vi "Load.vi"(8 "error in (no error)":errorcluster, 10 "Path":path, 11 "CNN in":refnum<class "CNN.lvclass">) -> (0 "error out":errorcluster, 3 "CNN out":refnum<class "CNN.lvclass">)   [LabVIEW 2016, in "CNN.lvclass"]
uses:
  CNN.lvclass
  CNN.lvclass/CNN.ctl
  <vilib>/Utility/file.llb/Read Delimited Spreadsheet (DBL).vi
panel:
  out "PFPC":i32[](array[numeric])
  out "all rows":dbl[][](array[numeric])
  out "size(s)":i32
  out "No Pre":i32[](array[numeric])
  out "Pre Ids":i32[](array[numeric])
  out "NoN":i32[](array[numeric])
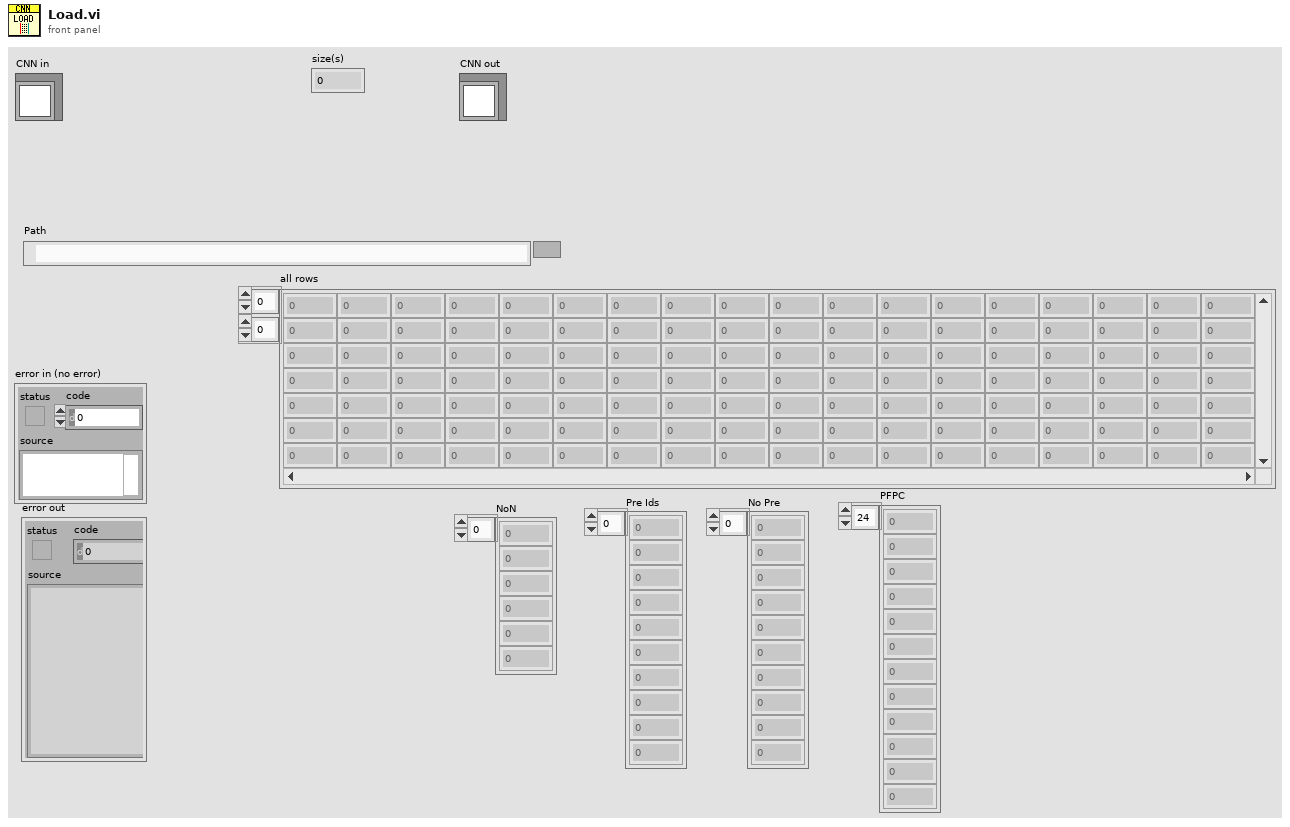
[diagram p1: front panel]
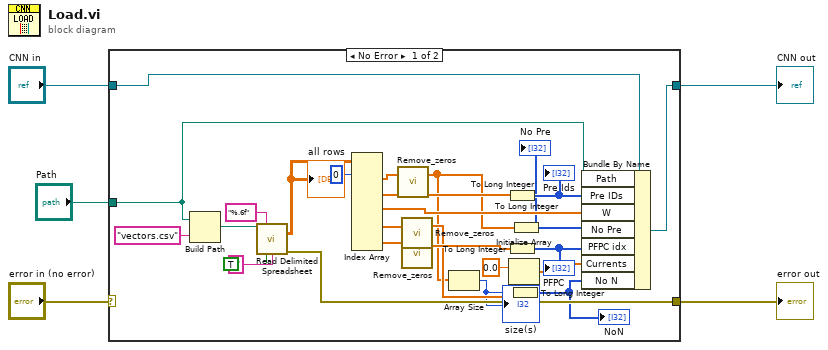
[diagram p0: block diagram]
diagram:
  n1 = case shown="No Error" "error in (no error)" {
    selector: "error in (no error)" -> [_ w32]
    tunnel: [w25 w32] -> w4
    tunnel: [w30 w33] -> w2
    tunnel: "CNN in" -> [w31 w33]
    tunnel: "Path" -> [w29 _]
    frame No Error {
      n2 = Build Path(base path=w29, name or relative path="vectors.csv") -> (appended path=w27:path)
      n3 = call-poly <vilib>:"Read Delimited Spreadsheet.vi"("file path (dialog if empty)"=w27, "format (%.3f)"="%.6f", "transpose? (F)"=TRUE, "delimiter (\\t)"="," ("delimiter (\\t)")) -> ("all rows"=w22:dbl[][], "error out"=w25:errorcluster)  [unwired: 6 in, 4 out]
      "all rows" <- w22
      n4 = Index Array(array=w22, index (row) #1=0 ("index (row)")) -> (element #1=w9:dbl[], element #2=w18:dbl[], element #3=w19:dbl[], element #4=w16:dbl[], element #5=w14:dbl[])  [unwired: 9 in]
      n5 = call "Remove_zeros.vi"("subarray in"=w9) -> ("subarray out"=w6:dbl[])  [unwired: 2 in]
      n6 = call "Remove_zeros.vi"("subarray in"=w16) -> ("subarray out"=w12:dbl[])  [unwired: 2 in]
      n7 = call "Remove_zeros.vi"("subarray in"=w14) -> ("subarray out"=w13:dbl[])  [unwired: 2 in]
      n8 = Array Size(array=w6) -> (size(s)=w8:i32)
      "size(s)" <- w8
      n9 = To Long Integer(number=w18) -> (32bit integer=w20:i32[])
      "Pre Ids" <- w20
      n10 = To Long Integer(number=w13) -> (32bit integer=w15:i32[])
      "PFPC" <- w15
      n11 = Initialize Array(0.0 ("element"), w8) -> (w11:dbl[])
      n12 = To Long Integer(number=w12) -> (32bit integer=w7:i32[])
      "NoN" <- w7
      n13 = To Long Integer(number=w6) -> (32bit integer=w17:i32[])
      "No Pre" <- w17
      n14 = Bundle By Name(cluster=w31, "Path"=w29, "Pre IDs"=w20, "W"=w19, "No Pre"=w17, "PFPC idx"=w15, "Currents"=w11, "No N"=w7) -> (w30:refnum<class "CNN.lvclass">)
    }
    frame Error {
    }
  }
  "error out" <- w4
  "CNN out" <- w2
